vi "Send XY Graph to Notebook (Optional).vi"(8 "error in (no error)":errorcluster, 9 "Send Graph to Notebook?":bool, 11 "XYGraph in":refnum<vi>) -> (0 "error out":errorcluster)   [LabVIEW 2019, in "Notebook.lvlib"]
uses:
  Notebook.lvlib
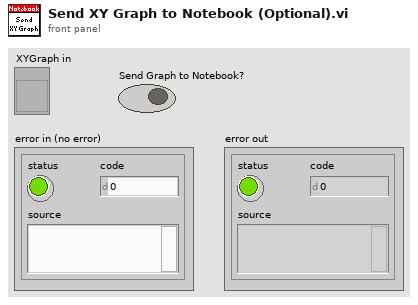
[diagram p1: front panel]
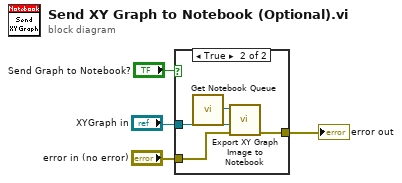
[diagram p0: block diagram]
diagram:
  n1 = case shown="True" "Send Graph to Notebook?" {
    tunnel: "error in (no error)" -> [w5 w9]
    tunnel: [w5 w8] -> w3
    tunnel: "XYGraph in" -> [_ w6]
    frame False {
    }
    frame True {
      n2 = call "Get Notebook Queue.vi"() -> ("Notebook Queue"=w7:refnum<queue>)  [unwired: 9 in]
      n3 = call "Export XY Graph Image to Notebook.vi"("Error In"=w9, "XYGraph Ref"=w6, "Notebook Q"=w7) -> ("Error Out"=w8:errorcluster)  [unwired: 8 in]
    }
  }
  "error out" <- w3
